vi "Get Link Type Value.vi"(10 "Override":u32=1, 11 "Link Types":T1) -> (3 "Link Type":u32)   [LabVIEW 2021, in "pcap Parse and Build.lvclass"]
uses:
  pcap Parse and Build.lvclass
  Typedef/Link Types.ctl
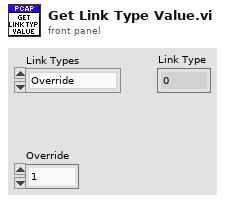
[diagram p1: front panel]
types:
  T1 = typedef "pcap Parse and Build.lvclass/Link Types.ctl" = enum16{"Override", "Ethernet", "Socket CAN", "I2C Linux"}
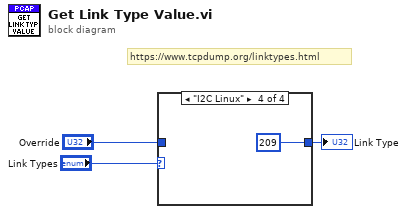
[diagram p0: block diagram]
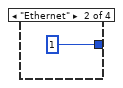
[diagram p3: hidden frame]
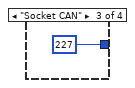
[diagram p4: hidden frame]
diagram:
  # "https://www.tcpdump.org/linktypes.html"
  n1 = case shown="\"I2C Linux\"" "Link Types" {
    tunnel: [w4 u32 1 u32 227 u32 209] -> w1
    tunnel: "Override" -> [w4 _ _ _]
    frame "Override" {
    }
    frame "Ethernet" {
    }
    frame "Socket CAN" {
    }
    frame "I2C Linux" {
    }
  }
  "Link Type" <- w1
